vi "test_OneSessTwoPinOneInstrTwoSiteReservation_CallNiDigitalGetConnections1PinMConnections_ReturnsTwoConnections.vi"(8 "error in":errorcluster) -> (0 "error out":errorcluster, 2 "result":string, 3 "pass":bool)   [LabVIEW 2020, in "MeasurementServerTests.lvlib"]
uses:
  MeasurementServerTests.lvlib
  Runtime/APIs/Session Management V1/Session Reservation/Connection.ctl
  Runtime/APIs/Session Management V1/Session Reservation/Session Reservation.lvclass
  03fc85e1-696b-4ece-a78b-f41470766ac0.vi
  a536e905-e99b-4ce6-9f7b-add65bd26abc.vi
  Runtime/Sessions/niDigital Sessions/Plug-In SDK niDigital Sessions.lvlib
  Runtime/Sessions/niDigital Sessions/Get Connections - 1Pin MConn.vi
  Runtime/Sessions/niDigital Sessions/Connection with Session.ctl
  b6660627-c938-49b4-8be7-8dfa183a54ed.vi
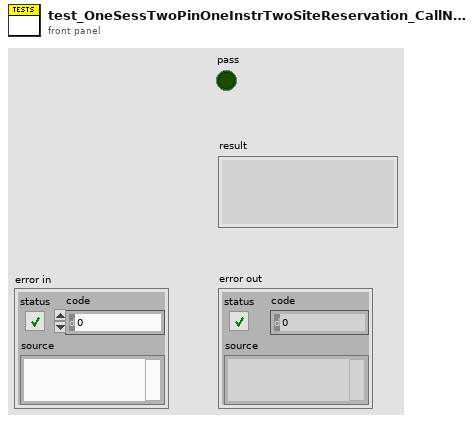
[diagram p1: front panel]
types:
  T1 = typedef "Plug-In SDK niDigital Sessions.lvlib/Connection with Session.ctl" = cluster{"connection":T2, "session":refnum<k15>}
  T2 = typedef "Plug-In SDK Session Management V1 API.lvlib/Session Reservation.lvclass/Connection.ctl" = cluster{"pin or relay name":string, "site":i32, "instrument type id":string, "channel":string}
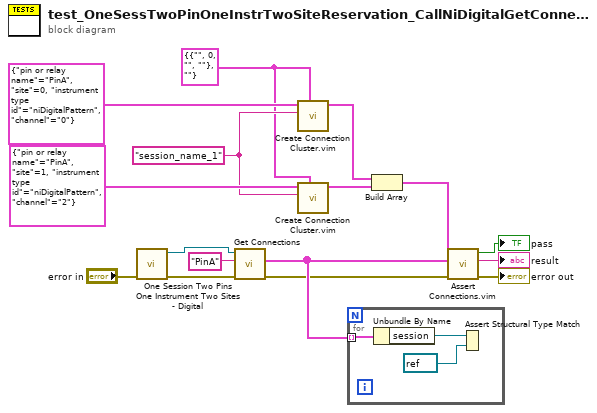
[diagram p0: block diagram]
diagram:
  w7 = T1 {"connection"={"pin or relay name"="", "site"=0, "instrument type id"="", "channel"=""}, "session"=""} ("connection with session")
  w12 = "session_name_1" ("session in")
  n1 = call "One Session Two Pins One Instrument Two Sites - Digital.vi"("error in"="error in") -> ("error out"=w4:errorcluster, "session reservation out"=w3:refnum<class "Session Reservation.lvclass">)  [unwired: 9 in]
  n2 = call-poly "Get Connections.vi"("error in"=w4, "pin or relay name"="PinA", "session reservation in"=w3) -> ("error out"=w2:errorcluster, "connections"=w5:T1[])  [unwired: 6 in, 1 out]
  n3 = call "Create Connection Cluster.vim"("connection type"=w7, "session in"=w12, "hardware independent connection in"=T2 {"pin or relay name"="PinA", "site"=0, "instrument type id"="niDigitalPattern", "channel"="0"} ("connection")) -> ("connection out"=w11:T1)  [unwired: 8 in]
  n4 = call "Create Connection Cluster.vim"("connection type"=w7, "session in"=w12, "hardware independent connection in"=T2 {"pin or relay name"="PinA", "site"=1, "instrument type id"="niDigitalPattern", "channel"="2"} ("connection")) -> ("connection out"=w10:T1)  [unwired: 8 in]
  n5 = for {
    tunnel: w5 -> [w17] mode=indexing
    n6 = Unbundle By Name(w17) -> ("session"=w19:refnum<k15>)
    n7 = Assert Structural Type Match(0:refnum<k15> refnum ("session"), 1:w19) -> ()
  }
  n8 = Build Array(w11, w10) -> (w9:T1[])
  n9 = call "Assert Connections.vim"("error in"=w2, "actual connections"=w5, "expected connections"=w9) -> ("error out"=→"error out":errorcluster, "result"=→"result":string, "pass"=→"pass":bool)  [unwired: 6 in]
